vi "PV HiLobe Set value settings.vi"(8 "error in (no error)":errorcluster, 9 "HiLobe Set value settings - Cluster":T1={"Parameter"=enum."Setpoint in speed setting mode [707]", "Parameter\nread only<->describe"=FALSE, "Setpoint in speed setting mode [707]"=75.0, "Unit adress"=1} caption="Operating adjustment - Cluster" {"Unit adress" min=1 max=255 step=1; "Setpoint in speed setting mode [707]" min=25.0 max=170.0 step=0.1 format="%.2f"}, 10 "Adress of unit":u16=1 min=1 max=999 step=1, 11 "VISA session":refnum<visa-resource-name>) -> (0 "error out":errorcluster, 2 "response (data)":string, 3 "dup VISA session":refnum<visa-resource-name>)   [LabVIEW 2021, in "Pfeiffer Vacuum.lvlib"]
doc: "There are 2 parameters available, only one of which can be enabled at a time. \n\nSetpoint in speed setting mode [707]\nRS-485 interface address [797]\n\nNote: The controls right of this one will set the appropriate values for the selected parameter. Any settings for an parameter that is not selected will be ignored. If a value is out of range, it will be changed to either the upper or the lower limit of the range."
uses:
  <instrlib>/Pfeiffer Vacuum/Pfeiffer Vacuum.lvlib
  <instrlib>/Pfeiffer Vacuum/Public/HiLobe/PV HiLobe Set value settings - Cluster.ctl
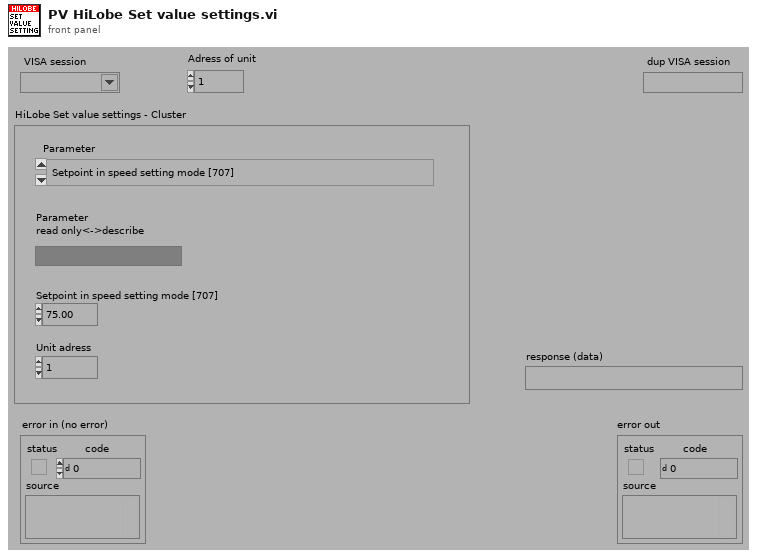
[diagram p1: front panel]
types:
  T1 = typedef "Pfeiffer Vacuum.lvlib/PV HiLobe Set value settings - Cluster.ctl" = cluster{"Parameter":enum16{"Setpoint in speed setting mode [707]", "RS-485 interface address [797]"}, "Parameter\nread only<->describe":bool, "Setpoint in speed setting mode [707]":dbl, "Unit adress":i16}
  T2 = enum16{"Setpoint in speed setting mode [707]", "RS-485 interface address [797]"}
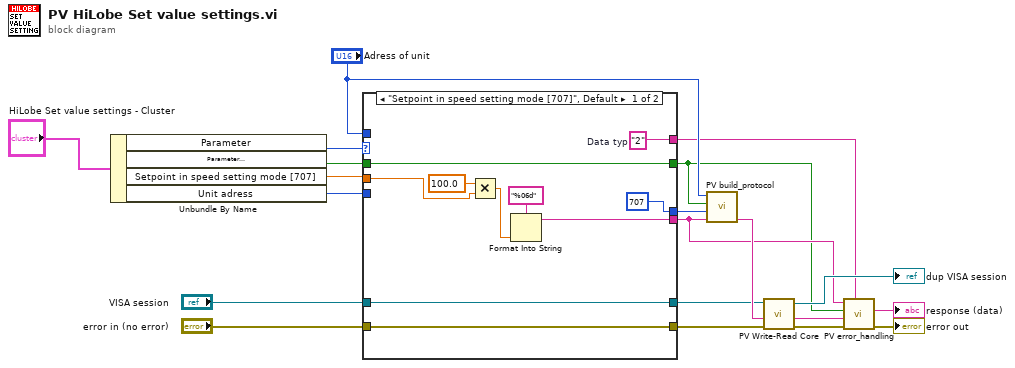
[diagram p0: block diagram]
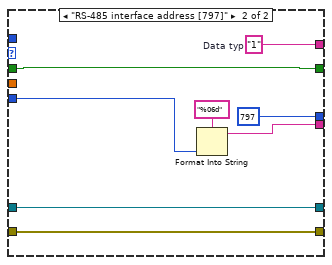
[diagram p2: hidden frame]
diagram:
  n1 = Unbundle By Name("HiLobe Set value settings - Cluster") -> ("Parameter"=w19:T2, "Parameter\nread only<->describe"=w18:bool, "Setpoint in speed setting mode [707]"=w3:dbl, "Unit adress"=w2:i16)
  n2 = case shown="\"Setpoint in speed setting mode [707]\", Default" w19 {
    tunnel: [u16 707 ("Parameter-number") u16 797 ("Parameter-number")] -> w20
    tunnel: [w22 w33] -> w8
    tunnel: [w25 w32] -> w6
    tunnel: w18 -> [w25 w32]
    tunnel: w3 -> [w21 _]
    tunnel: [w24 w31] -> w7
    tunnel: "VISA session" -> [w30 w38]
    tunnel: [w30 w38] -> w13
    tunnel: "Adress of unit" -> [_ _]
    tunnel: "error in (no error)" -> [w29 w37]
    tunnel: [w29 w37] -> w12
    tunnel: w2 -> [_ w35]
    frame "Setpoint in speed setting mode [707]", Default {
      w24 = "2"  # Data typ
      n3 = Multiply(x=100.0, y=w21) -> (x*y=w27:dbl)
      n4 = Format Into String(format string="%06d" ("Format-String"), w27) -> (resulting string=w22:string)  [unwired: 2 in, 1 out]
    }
    frame "RS-485 interface address [797]" {
      w31 = "1"  # Data typ
      n5 = Format Into String(format string="%06d" ("Format-String"), w35) -> (resulting string=w33:string)  [unwired: 2 in, 1 out]
    }
  }
  n6 = call <instrlib>:"PV build_protocol.vi"("Data"=w8, "Parameter-number"=w20, "parameter\nread<->describe"=w6, "Adress"="Adress of unit") -> ("output"=w14:string)  [unwired: 3 in]
  n7 = call <instrlib>:"PV Write-Read Core.vi"("error in"=w12, "Write data in"=w14, "VISA session"=w13) -> ("error out"=w10:errorcluster, "response (data) out"=w11:string, "dup VISA session"=→"dup VISA session":refnum<visa-resource-name>)  [unwired: 2 in]
  n8 = call <instrlib>:"PV error_handling.vi"("Data Typ in"=w7, "error in"=w10, "response (data) in"=w11, "Parameter\nread only<->describe"=w6, "data in"=w8) -> ("error out"=→"error out":errorcluster, "Data out"=→"response (data)":string)  [unwired: 4 in, 1 out]
